vi "UpdateStepResult.vi"(8 "error in (no error)":errorcluster, 10 "Result":T1, 11 "Index":T3) -> (0 "error out":errorcluster, 3 "Update?":bool)   [LabVIEW 2016, in "SeqProcessor.lvlib"]
uses:
  SeqProcessor.lvlib
  controls/StepIndex.ctl
  controls/StepResult.ctl
  controls/StepStatus.ctl
  controls/NormalStep.ctl
  controls/StepAction.ctl
  controls/JumpStep.ctl
  controls/ConditionalStep.ctl
  controls/ParallelStep.ctl
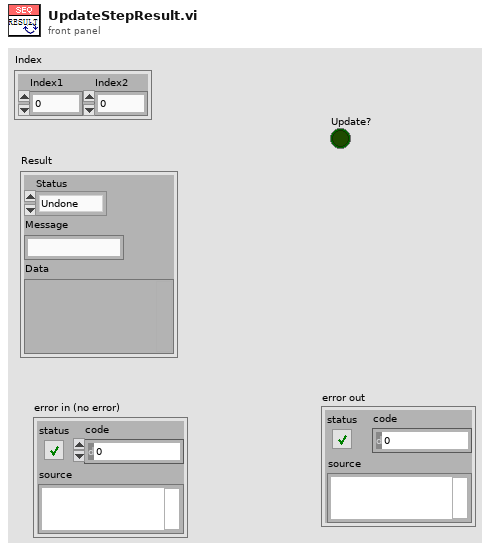
[diagram p1: front panel]
types:
  T1 = typedef "SeqProcessor.lvlib/StepResult.ctl" = cluster{"Status":T2, "Message":string, "Data":variant}
  T2 = typedef "SeqProcessor.lvlib/StepStatus.ctl" = enum16{"Undone", "Finish", "Error"}
  T3 = typedef "SeqProcessor.lvlib/StepIndex.ctl" = cluster{"Index1":u32, "Index2":u32}
  T4 = typedef "SeqProcessor.lvlib/Step.ctl" = cluster{"Type":T5, "Step":variant}
  T5 = typedef "SeqProcessor.lvlib/StepType.ctl" = enum16{"Normal", "Parallel", "Conditional", "Jump"}
  T6 = typedef "SeqProcessor.lvlib/NormalStep.ctl" = cluster{"Action":T7, "Result":T1}
  T7 = typedef "SeqProcessor.lvlib/StepAction.ctl" = cluster{"Action":string, "Process":string, "Data":variant, "Condition":variant}
  T8 = typedef "SeqProcessor.lvlib/JumpStep.ctl" = cluster{"Action":T7, "Jump":i32, "Result":T1}
  T9 = typedef "SeqProcessor.lvlib/ConditionalStep.ctl" = cluster{"Action":T7, "Result":T1}
  T10 = typedef "SeqProcessor.lvlib/ParallelStep.ctl" = T6[]
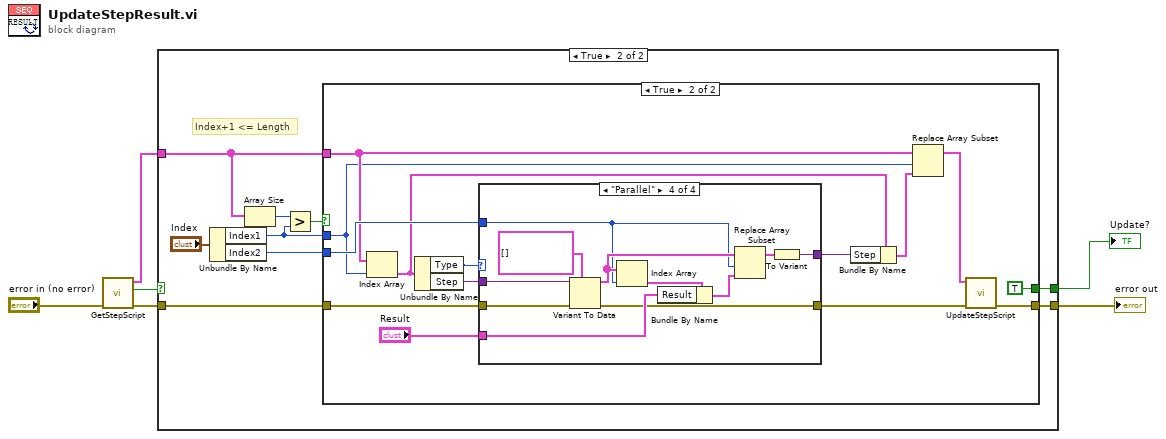
[diagram p0: block diagram]
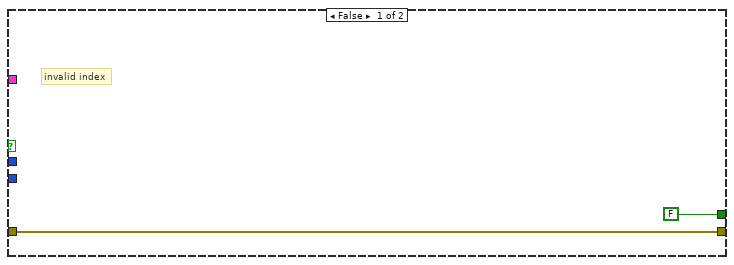
[diagram p3: hidden frame]
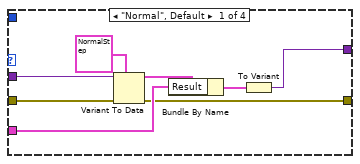
[diagram p4: hidden frame]
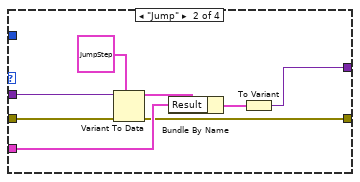
[diagram p5: hidden frame]
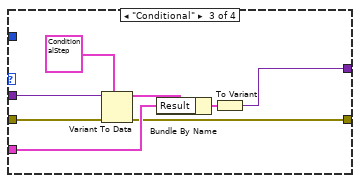
[diagram p6: hidden frame]
diagram:
  n1 = call "GetStepScript.vi"("error in (no error)"="error in (no error)") -> ("error out"=w4:errorcluster, "found"=w5:bool, "StepScript"=w3:T4[])  [unwired: 8 in]
  n2 = case shown="True" w5 {
    selector: w5 -> [w7 _]
    tunnel: w4 -> [w8 w17]
    tunnel: w3 -> [_ w15]
    tunnel: [w8 w10] -> w2
    tunnel: [w7 w9] -> w1
    frame False {
    }
    frame True {
      # "Index+1 <= Length"
      n3 = Unbundle By Name("Index") -> ("Index1"=w13:u32, "Index2"=w11:u32)
      n4 = Array Size(array=w15) -> (size(s)=w14:i32)
      n5 = Greater?(x=w14, y=w13) -> (0:w12:bool)
      n6 = case shown="True" w12 {
        tunnel: w17 -> [w19 w31]
        tunnel: w15 -> [_ w25]
        tunnel: w13 -> [_ w23]
        tunnel: w11 -> [_ w29]
        tunnel: [w19 w21] -> w10
        tunnel: [FALSE TRUE] -> w9
        frame False {
          # "invalid index"
        }
        frame True {
          n7 = Index Array(array=w25, index=w23) -> (element=w24:T4)
          n8 = Unbundle By Name(w24) -> ("Type"=w33:T5, "Step"=w32:variant)
          n9 = case shown="\"Parallel\"" w33 {
            tunnel: w32 -> [w41 w49 w57 w68]
            tunnel: w31 -> [w39 w48 w56 w67]
            tunnel: "Result" -> [w37 w46 w54 w66]
            tunnel: [w35 w44 w52 w65] -> w28
            tunnel: w29 -> [_ _ _ w61]
            tunnel: [w34 w43 w51 w58] -> w26
            frame "Normal", Default {
              n10 = Variant To Data(error in=w39, type=T6 {"Action"={"Action"="", "Process"="", "Data"=variant, "Condition"=variant(bool FALSE)}, "Result"={"Status"=enum."Undone", "Message"="", "Data"=variant}} ("NormalStep"), Variant=w41) -> (data=w38:T6, error out=w35:errorcluster)
              n11 = Bundle By Name(cluster=w38, "Result"=w37) -> (w36:T6)
              n12 = To Variant(anything=w36) -> (Variant=w34:variant)
            }
            frame "Jump" {
              n13 = Variant To Data(error in=w48, type=T8 {"Action"={"Action"="", "Process"="", "Data"=variant, "Condition"=variant(bool FALSE)}, "Jump"=0, "Result"={"Status"=enum."Undone", "Message"="", "Data"=variant}} ("JumplStep"), Variant=w49) -> (data=w47:T8, error out=w44:errorcluster)
              n14 = Bundle By Name(cluster=w47, "Result"=w46) -> (w45:T8)
              n15 = To Variant(anything=w45) -> (Variant=w43:variant)
            }
            frame "Conditional" {
              n16 = Variant To Data(error in=w56, type=T9 {"Action"={"Action"="", "Process"="", "Data"=variant, "Condition"=variant(bool FALSE)}, "Result"={"Status"=enum."Undone", "Message"="", "Data"=variant}} ("ConditionlStep"), Variant=w57) -> (data=w55:T9, error out=w52:errorcluster)
              n17 = Bundle By Name(cluster=w55, "Result"=w54) -> (w53:T9)
              n18 = To Variant(anything=w53) -> (Variant=w51:variant)
            }
            frame "Parallel" {
              n19 = Variant To Data(error in=w67, type=T10 [] ("ParallelStep"), Variant=w68) -> (data=w62:T10, error out=w65:errorcluster)
              n20 = Index Array(array=w62, index=w61) -> (element=w63:T6)
              n21 = Bundle By Name(cluster=w63, "Result"=w66) -> (w60:T6)
              n22 = Replace Array Subset(array=w62, new element=w60, index=w61) -> (w59:T10)
              n23 = To Variant(anything=w59) -> (Variant=w58:variant)
            }
          }
          n24 = Bundle By Name(cluster=w24, "Step"=w26) -> (w27:T4)
          n25 = Replace Array Subset(array=w25, new element=w27, index=w23) -> (w22:T4[])
          n26 = call "UpdateStepScript.vi"("error in (no error)"=w28, "StepScript"=w22) -> ("error out"=w21:errorcluster)  [unwired: 9 in]
        }
      }
    }
  }
  "error out" <- w2
  "Update?" <- w1
